vi "RX OOB Test Cases.vi"() -> (0 "error out":errorcluster, 2 "status":string, 3 "pass":bool)   [LabVIEW 2021]
uses:
  OOB_Rx/Typedef/gRPC to Main Command Data.ctl
  CIF-LVCore/src/CIFUtilities/CIFOutOfBand/CIFOutOfBand.lvclass/CIFOutOfBand.ctl
  OOB_Rx/Typedef/OOB Commands.ctl
  OOB_Rx/Private/Command Settings.vi
  CIF-LVCore/src/CIFUtilities/CIFOutOfBand/Accessors/Write Local OOB Data.vi
  CIF-LVCore/src/CIFUtilities/CIFOutOfBand/Write OOB DVR.vi
  CIF-LVCore/src/CIFUtilities/CIFOutOfBand/Utilities/Command to Bitwise Command.vi
  CIF-LVCore/src/CIFUtilities/CIFOutOfBand/Accessors/Read Local OOB Data.vi
  CIF-LVCore/src/CIFUtilities/CIFOutOfBand/Read OOB DVR.vi
  OOB_Rx/Private/Read Payload.vi
  OOB_Rx/TemplateOOB_Rx.lvclass
  D:/dev/CIF-LVCore/src/CIFUtilities/CIFOutOfBand/CIFOutOfBand.lvclass
  CIF-LVCore/src/CIFUtilities/CIFOutOfBand/Init OOB.vi
  CIF-LVCore/src/CIFUtilities/CIFOutOfBand/CIFOutOfBand.lvclass
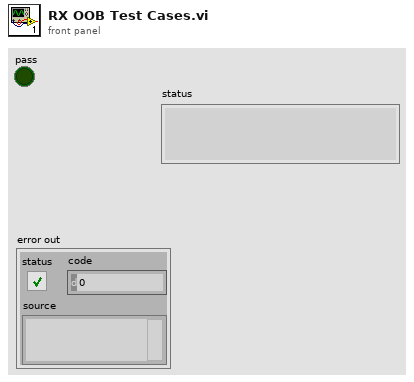
[diagram p1: front panel]
types:
  T1 = typedef "TemplateOOB_Rx.lvclass/gRPC to Main Command Data.ctl" = cluster{"Cmd 1 Data":i32}
  T2 = typedef "TemplateOOB_Rx.lvclass/OOB Commands.ctl" = enum8{"Command 1"}
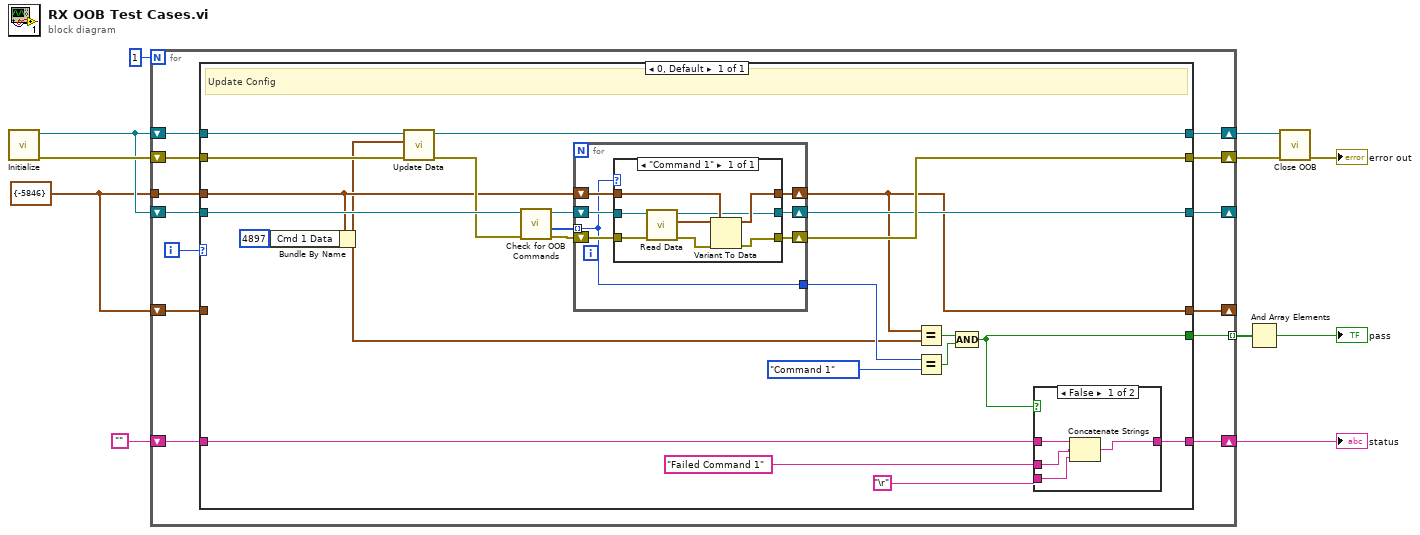
[diagram p0: block diagram]
diagram:
  w1 = T1 {"Cmd 1 Data"=-5846} ("Data")
  n1 = call "Initialize.vi"() -> ("error out"=w3:errorcluster, "CutomOOB_Rx out"=w2:refnum<class "TemplateOOB_Rx.lvclass">)  [unwired: 10 in]
  n2 = for {
    N: 1 -> [_]
    tunnel: [w24] -> w9 mode=indexing
    tunnel: w1 -> [w22]
    shift-right: [w21] -> w10
    shift-left: w3 -> [w23]
    shift-right: [w12] -> w11
    shift-left: w2 -> [w13]
    shift-right: [w18] -> _
    shift-left: w2 -> [w19]
    shift-right: [w17] -> _
    shift-left: w1 -> [w16]
    shift-right: [w14] -> w6
    shift-left: "" -> [w15]
    i -> [w20]
    n3 = case shown="0, Default" w20 {
      tunnel: [w35] -> w24
      tunnel: w23 -> [w31]
      tunnel: w22 -> [w29]
      tunnel: w13 -> [w27]
      tunnel: [w47] -> w21
      tunnel: [w32] -> w12
      tunnel: w19 -> [w41]
      tunnel: [w46] -> w18
      tunnel: [w28] -> w17
      tunnel: w16 -> [_]
      tunnel: w15 -> [w45]
      tunnel: [w44] -> w14
      frame 0, Default {
        # "Update Config"
        n4 = Bundle By Name(cluster=w29, "Cmd 1 Data"=4897 ("Numeric")) -> (w25:T1)
        n5 = call "Update Data.vi"("error in"=w31, "Data"=w25, "CutomOOB_Rx in"=w27) -> ("error out"=w30:errorcluster, "CutomOOB_Rx out"=w32:refnum<class "TemplateOOB_Rx.lvclass">)  [unwired: 7 in]
        n6 = call "Check for OOB Commands.vi"("error in (no error)"=w30, "CoreOOB_Rx in"=w41) -> ("error out"=w40:errorcluster, "Commands"=w38:T2[], "CoreOOB_Rx out"=w39:refnum<class "TemplateOOB_Rx.lvclass">)  [unwired: 6 in, 1 out]
        n7 = for {
          tunnel: w38 -> [w48] mode=indexing
          shift-right: [w49] -> w28
          shift-left: w29 -> [w54]
          shift-right: [w53] -> w47
          shift-left: w40 -> [w51]
          shift-right: [w52] -> w46
          shift-left: w39 -> [w50]
          tunnel: [w48] -> w34
          n8 = case shown="\"Command 1\"" w48 {
            tunnel: w50 -> [w58]
            tunnel: w51 -> [w59]
            tunnel: [w57] -> w52
            tunnel: w54 -> [w62]
            tunnel: [w61] -> w53
            tunnel: [w60] -> w49
            frame "Command 1" {
              n9 = call "Read Data.vi"("error in"=w59, "CutomOOB_Rx in"=w58) -> ("error out"=w55:errorcluster, "Data"=w56:T1, "CutomOOB_Rx out"=w57:refnum<class "TemplateOOB_Rx.lvclass">)  [unwired: 7 in]
              n10 = Variant To Data(error in=w55, type=w62, Variant=w56) -> (data=w60:T1, error out=w61:errorcluster)
            }
          }
        }
        n11 = Equal?(x=w28, y=w25) -> (x = y?=w37:bool)
        n12 = Equal?(x=w34, y=OOB_Commands."Command 1") -> (x = y?=w36:bool)
        n13 = Compound Arithmetic op=AND(w37, w36) -> (w35:bool)
        n14 = case shown="False" w35 {
          tunnel: w45 -> [w66 w67]
          tunnel: [w63 w67] -> w44
          tunnel: "Failed Command 1" -> [w65 _]
          tunnel: "\r" -> [w64 _]
          frame False {
            n15 = Concatenate Strings(w66, w65, w64) -> (w63:string)
          }
          frame True {
          }
        }
      }
    }
  }
  "status" <- w6
  n16 = And Array Elements(Boolean array=w9) -> (logical AND=→"pass":bool)
  n17 = call "Close OOB.vi"("error in"=w10, "OOB in"=w11) -> ("error out"=→"error out":errorcluster)  [unwired: 9 in]
